vi "Single Tone Measurements.vi"() -> ()   [LabVIEW 2022 SP3]
uses:
  <vilib>/PDM Acquisition Toolkit/host/Classes/Session/Controls/Logic Levels.ctl
  <vilib>/PDM Acquisition Toolkit/shared/controls/decimation order.ctl
  source/shared/measurements/controls/single tone microphone measurements.ctl
  <vilib>/addons/_NISVFA/_Generation/Signal Generation/SV Signal/sv_System Timing Model.ctl
  <vilib>/PDM Acquisition Toolkit/host/Classes/Tasks/PDM Tasks/Controls/Acquisition Mode.ctl
  <vilib>/PDM Acquisition Toolkit/shared/controls/clock mode.ctl
  <vilib>/PDM Acquisition Toolkit/host/API/Controls/PDM Digital Start Trigger Cluster.ctl
  <vilib>/PDM Acquisition Toolkit/shared/controls/PXI trigger lines.ctl
  <vilib>/PDM Acquisition Toolkit/shared/controls/trigger polarity.ctl
  source/shared/Stop Variable Action.ctl
  source/shared/measurements/controls/audio filter settings.ctl
  class-d-amplifier/source/shared/controls/weighting filter.ctl
  class-d-amplifier/source/shared/controls/highpass filter.ctl
  class-d-amplifier/source/shared/controls/lowpass filter.ctl
  source/shared/measurements/controls/units settings - mic.ctl
  source/shared/measurements/controls/measurement units.ctl
  source/shared/measurements/controls/single tone microphone measurement settings.ctl
  <vilib>/DAQmx/read.llb/DAQmx Read (Analog Wfm 1Chan NSamp).vi
  <vilib>/DAQmx/write.llb/DAQmx Write (Analog Wfm 1Chan NSamp).vi
  <vilib>/addons/_NISVFA/_Generation/Signal Generation/SV Sinusoid/SV Sinusoid.lvclass
  C:/Program Files/NI/LVAddons/nisvt/1/vi.lib/addons/_NISVFA/_Generation/Signal Generation/SV Signal/SV Signal.lvclass
  <vilib>/PDM Acquisition Toolkit/host/API/Public/Create Tasks/Create PDM Input Task.vi
  <vilib>/PDM Acquisition Toolkit/host/API/Public/Configure/Timing/Configure Timing - PDM Input.vi
  <vilib>/PDM Acquisition Toolkit/host/API/Public/Configure/PDM Channel/Configure Microphone Sensitivity DBFS.vi
  <vilib>/PDM Acquisition Toolkit/host/API/Public/Configure/Triggering/Configure PDM Trigger (Digital Edge).vi
  <vilib>/PDM Acquisition Toolkit/host/API/Public/Read/Read PCM Waveform.vi
  <vilib>/Waveform/WDTOps.llb/WDT Waveform Duration DBL.vi
  <vilib>/Waveform/WDTOps.llb/WDT Get Waveform Subset DBL.vi
  <vilib>/addons/_NISVFA/_Generation/Signal Generation/SV Sinusoid/Configure Sine.vi
  <vilib>/DAQmx/create/channels.llb/DAQmx Create Channel (AO-Voltage-Basic).vi
  <vilib>/DAQmx/configure/timing.llb/DAQmx Timing (Sample Clock).vi
  <vilib>/DAQmx/configure/events/hardwareSignals.llb/DAQmx Export Signal (Most Signals).vi
  <vilib>/addons/_NISVFA/_Generation/Signal Generation/SV Signal/Write Sample Rate.vi
  <vilib>/addons/_NISVFA/_Generation/Signal Generation/SV Signal/Write System Timing Model.vi
  <vilib>/addons/_NISVFA/_Generation/Signal Generation/SV Signal/Write Ramp Parameters.vi
  <vilib>/DAQmx/create/channels.llb/DAQmx Create Channel (AI-Sound Pressure-Microphone).vi
  <vilib>/DAQmx/configure/trigger.llb/DAQmx Start Trigger (Digital Edge).vi
  <vilib>/DAQmx/miscellaneous.llb/DAQmx Fill In Error Info.vi
  <vilib>/addons/Sound and Vibration/svt_Level/SVL Leq Sound Level (1 Ch).vi
  <vilib>/PDM Acquisition Toolkit/host/API/Public/Clear/Clear PDM Input Task.vi
  <vilib>/addons/_NISVFA/_Generation/Signal Generation/SV Signal/SV Signal.lvclass
  <resource>/objmgr/daqmx.rc
  <vilib>/addons/Sound and Vibration/svt_Level/SoundVib_SoundLevel.lvlib
  <vilib>/PDM Acquisition Toolkit/host/API/PDM Acquisition Toolkit.lvlib
  <vilib>/PDM Acquisition Toolkit/host/Classes/Tasks/PDM Tasks/PDM Task.lvclass
  <vilib>/PDM Acquisition Toolkit/shared/PDM Shared.lvlib
  <vilib>/PDM Acquisition Toolkit/host/Classes/Session/DecoderSession.lvclass
panel:
  out "measurements":T1
  in  "Tab Control":enum32{"Time Domain", "Spectrum"}(tab)
  out "Waveform Graph":waveform(dbl)[](graph)
  out "Spectrum":cluster{"x0":dbl, "dx":dbl, "magnitude":dbl[]}[](graph)
  out "microphone sensitivity (dBFS)":dbl
  out "Ref Mic Sound Level":dbl format="%.2f"
  out "Error Out":errorcluster
  out "Actual PCM Clock Rate":dbl=47999.99987881165 format="%#_6p"
  out "Actual PDM Clock Rate":dbl=3071999.9922439456 format="%#_6p"
  out "Digital Mic Sound Level":dbl=102.39991597507856 format="%.2f"
  in  "Microphone Sensitivity (dBFS)":dbl=-26.0 format="%#_13g"
  in  "PDM Clock Rate":dbl=3072000.0 format="%#_6p"
  in  "Decimation Factor":T2=64 items=["24"=24, "32"=32, "48"=48, "64"=64, "96"=96, "128"=128]
  in  "Logic Level":T3
  in  "PDM Channels":string="PXI1Slot5\\PDMi 0"
  in  "output voltage ratio":dbl=3.39 format="%#_g Pa/V"
  in  "amplitude":dbl=94.0 format="%.2p dBSPL"
  in  "sensor sensitivity [mV/Pa]":dbl=50.0
  in  "physical channel":tag="PXI1Slot2/ai0"
  in  "output channels":tag="PXI1Slot2/ao0"
  in  "frequency":dbl=1000.0 format="%#_g Hz"
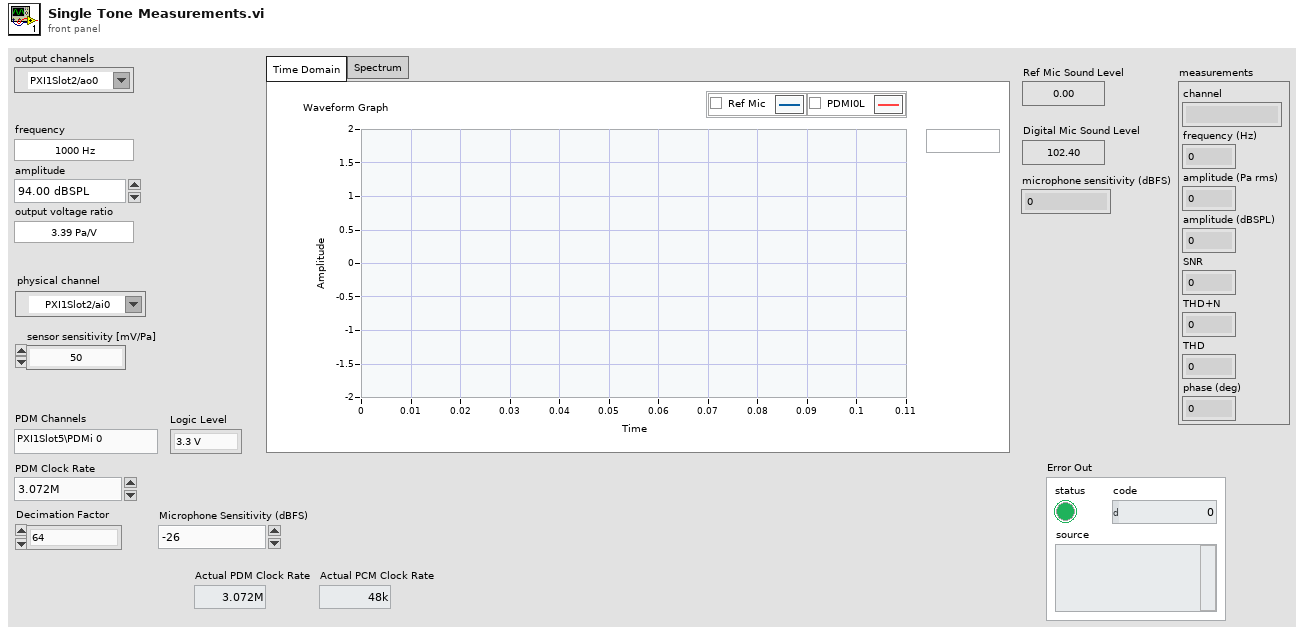
[diagram p1: front panel]
types:
  T1 = typedef "single tone microphone measurements.ctl" = cluster{"channel":string, "frequency (Hz)":dbl, "amplitude (Pa rms)":dbl, "amplitude (dBSPL)":dbl, "SNR":dbl, "THD+N":dbl, "THD":dbl, "phase (deg)":dbl}
  T2 = typedef "PDM Shared.lvlib/decimation order.ctl" = u16
  T3 = typedef "PDM Acquisition Class Library.lvlib/DecoderSession.lvclass/Logic Levels.ctl" = enum16{"3.3 V", "1.8 V", "1.2 V"}
  T4 = typedef "single tone microphone measurement settings.ctl" = cluster{"Band start":dbl, "Band stop":dbl, "Frequency":dbl}
  T5 = typedef "units settings - mic.ctl" = cluster{"SNR units":T6, "THD+N units":T6, "THD units":T6}
  T6 = typedef "measurement units.ctl" = enum32{"dB", "%", "x/y"}
  T7 = typedef "audio filter settings.ctl" = cluster{"weighting filter":T8, "highpass filter":T9, "lowpass filter ":T10}
  T8 = typedef "weighting filter.ctl" = enum32{"Linear", "A-weighting", "B-weighting", "C-weighting"}
  T9 = typedef "highpass filter.ctl" = enum32{"DC", "AC"}
  T10 = typedef "lowpass filter.ctl" = enum32{"No filter", "AES17 20kHz", "AES17 40kHz"}
  T11 = typedef "Stop Variable Action.ctl" = enum16{"Reset", "Check", "Stop"}
  T12 = typedef "PDM Acquisition Toolkit.lvlib/PDM Digital Start Trigger Cluster.ctl" = cluster{"source":T13, "polarity":T14}
  T13 = typedef "PDM Shared.lvlib/PXI trigger lines.ctl" = enum16{"PXI_Trig0", "PXI_Trig1", "PXI_Trig2", "PXI_Trig3", "PXI_Trig4", "PXI_Trig5", "PXI_Trig6", "PXI_Trig7"}
  T14 = typedef "PDM Shared.lvlib/trigger polarity.ctl" = enum16{"Rising Edge", "Falling Edge"}
  T15 = typedef "PDM Shared.lvlib/clock mode.ctl" = enum16{"divided clock", "DDS"}
  T16 = typedef "PDM Acquisition Class Library.lvlib/PDM Task.lvclass/Acquisition Mode.ctl" = enum16{"Finite", "Continuous"}
  T17 = typedef "SV Signal.lvclass/sv_System Timing Model.ctl" = i64
  T18 = cluster{"profile":enum16{"Linear", "Half cosine"}, "durations [s]":cluster{"ramp-up":dbl, "transition":dbl, "ramp-down":dbl}}
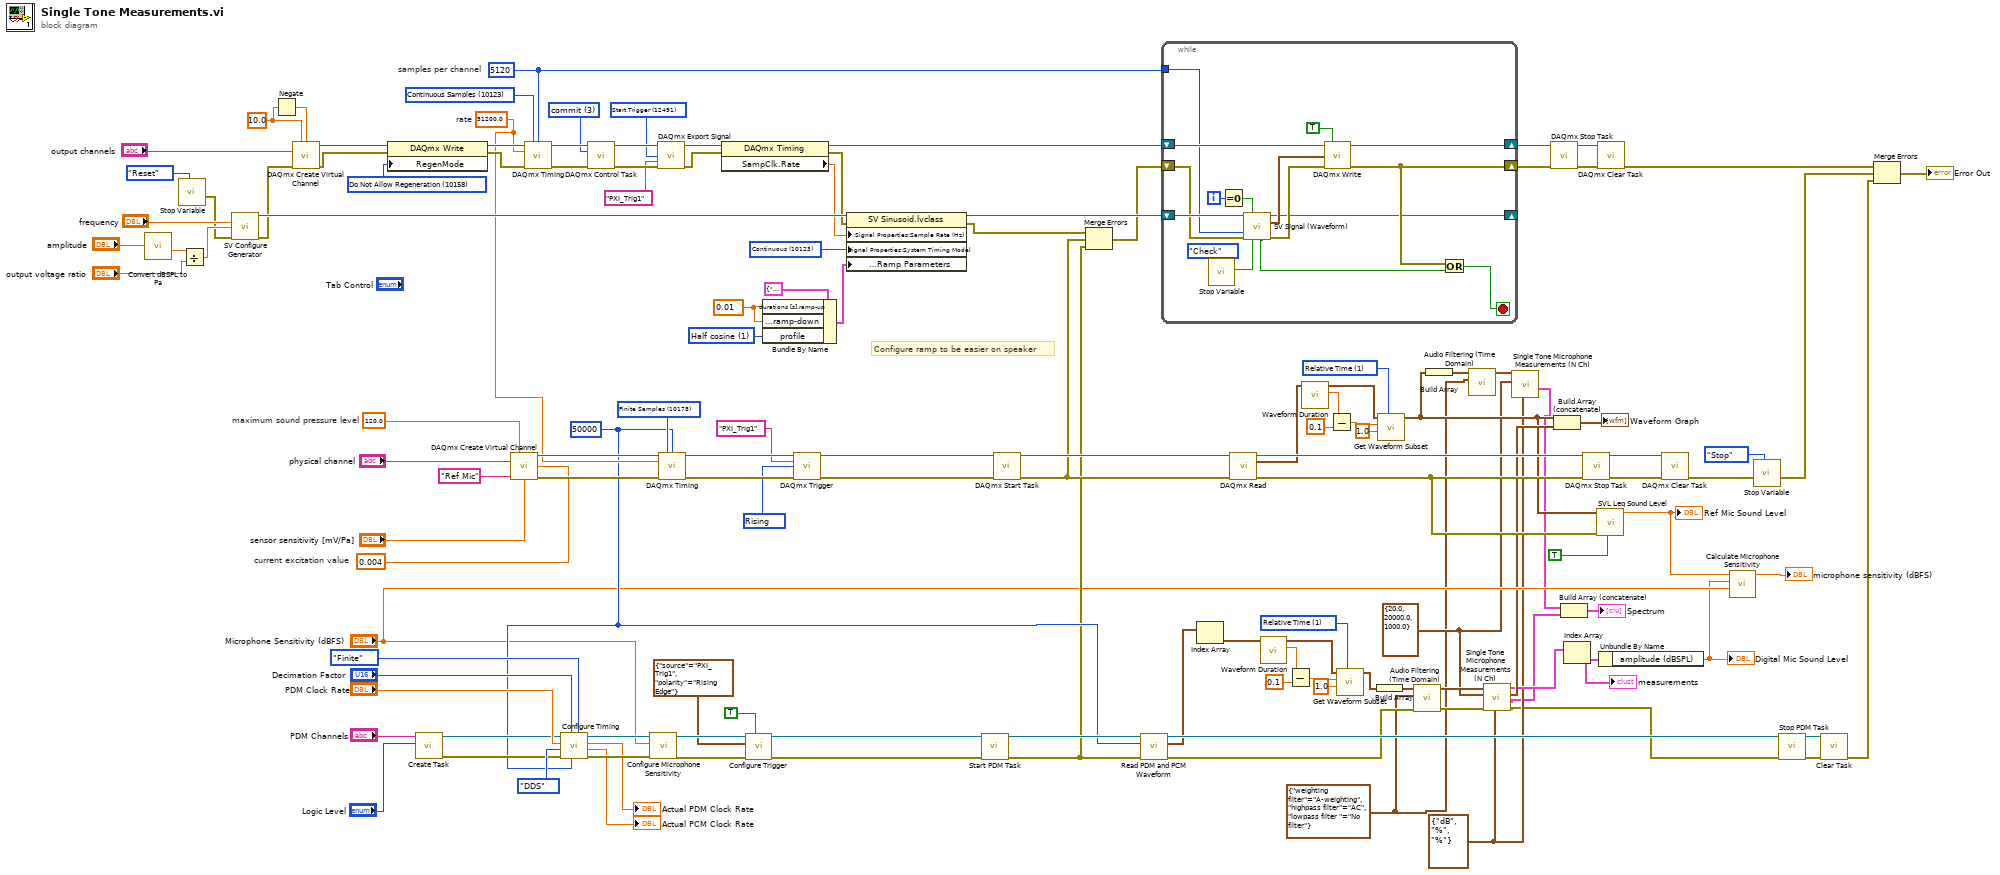
[diagram p0: block diagram]
diagram:
  w7 = T4 {"Band start"=20.0, "Band stop"=20000.0, "Frequency"=1000.0} ("measurement settings")
  w5 = T5 {"SNR units"=enum."dB", "THD+N units"=enum."%", "THD units"=enum."%"} ("units settings")
  w6 = T7 {"weighting filter"=enum."A-weighting", "highpass filter"=enum."AC", "lowpass filter "=enum."No filter"} ("filter settings")
  w38 = u16 1 items=["Samples", "Relative Time"] ("start/duration format")
  w44 = u16 1 items=["Samples", "Relative Time"] ("start/duration format")
  w61 = 50000 ("samples per channel")
  w62 = 10280 items=["Rising"=10280, "Falling"=10171] ("edge")
  w69 = 12491 items=["AI Convert Clock"=12484, "10MHz Reference Clock"=12536, "20MHz Timebase Clock"=12486, "Sample Clock"=12487, "Advance Trigger"=12488, "Reference Trigger"=12490, "Start Trigger"=12491, "Advance Complete Event"=12492, "AI Hold Complete Event"=12493, "Counter Output Event"=12494, "Change Detection Event"=12511, "Watchdog Timer Expired Event"=12512] ("signal")
  w74 = 3 items=["verify"=2, "reserve"=4, "commit"=3, "unreserve"=5, "abort"=6] ("action")
  w131 = 0.01 ("ramp duration")
  w129 = u16 1 items=["Linear", "Half cosine"] ("ramp profile")
  w109 = 0.004  # current excitation value
  w113 = 120.0  # maximum sound pressure level
  w115 = 10178 items=["Finite Samples"=10178, "Continuous Samples"=10123] ("sample mode")
  w122 = 10158 items=["Allow Regeneration"=10097, "Do Not Allow Regeneration"=10158] ("RegenMode")
  w125 = 10.0 ("maximum value")
  w102 = 5120  # samples per channel
  w126 = 10123 items=["Finite Samples"=10178, "Continuous Samples"=10123, "Hardware Timed Single Point"=12522] ("sample mode")
  w105 = 51200.0  # rate
  w128 = T17 10123 items=["Finite"=10178, "-"=-1, "Continuous"=10123, "-"=-2, "Settled"=110123, "Averaged"=210123, "Discrete Sweep"=310123, "Continuous Sweep"=410123] ("System Timing Model")
  # "Configure ramp to be easier on speaker"
  n1 = call "Convert dBSPL to Pa.vi"("dB SPL"="amplitude") -> ("Pa pk"=w95:dbl)  [unwired: 9 in, 1 out]
  n2 = call "Stop Variable.vi"("action"=Stop_Variable_Action."Reset") -> ("error out"=w35:errorcluster)  [unwired: 9 in, 1 out]
  n3 = Divide(x=w95, y="output voltage ratio") -> (x/y=w94:dbl)
  n4 = call-poly <vilib>:"SV Configure Generator.vi"("frequency (Hz)"="frequency", "amplitude"=w94, "error in (no error)"=w35) -> ("signal configuration"=w133:refnum<class "SV Sinusoid.lvclass">, "error out"=w123:errorcluster)  [unwired: 11 in]
  n5 = Negate(x=w125) -> (-x=w124:dbl)
  n6 = call-poly <vilib>:"DAQmx Create Virtual Channel.vi"("maximum value"=w125, "minimum value"=w124, "physical channels"="output channels", "error in"=w123) -> ("task out"=w121:refnum<k21>, "error out"=w119:errorcluster)  [unwired: 10 in]
  n7 = property class="DAQmx Write"(reference=w121, error in=w119, "RegenMode"=w122) -> (reference out=w120:refnum<k21>, error out=w118:errorcluster)
  n8 = call-poly <vilib>:"Create Task.vi"("logic level"="Logic Level", "channel list"="PDM Channels") -> ("error out"=w80:errorcluster, "PDM input task out"=w81:refnum<data-value>)  [unwired: 8 in]
  n9 = call-poly <vilib>:"DAQmx Create Virtual Channel.vi"("maximum sound pressure level"=w113, "physical channels"="physical channel", "name to assign"="Ref Mic", "current excitation value"=w109, "microphone sensitivity"="sensor sensitivity [mV/Pa]") -> ("task out"=w111:refnum<k21>, "error out"=w110:errorcluster)  [unwired: 9 in]
  n10 = call-poly <vilib>:"DAQmx Timing.vi"("task/channels in"=w120, "sample mode"=w126, "samples per channel"=w102, "rate"=w105, "error in"=w118) -> ("task out"=w76:refnum<k21>, "error out"=w75:errorcluster)  [unwired: 9 in]
  n11 = call-poly <vilib>:"Configure Timing.vi"("acquisition mode"=Acquisition_Mode."Finite" ("Acquisition Mode"), "number of PCM samples"=w61, "decimation factor"="Decimation Factor", "error in"=w80, "clock mode"=clock_mode."DDS" ("Clock Type"), "PDM clock rate"="PDM Clock Rate", "PDM input task in"=w81) -> ("error out"=w84:errorcluster, "actual PCM clock rate"=→"Actual PCM Clock Rate":dbl, "actual PDM clock rate"=→"Actual PDM Clock Rate":dbl, "PDM input task out"=w85:refnum<data-value>)  [unwired: 1 in]
  n12 = call <vilib>:"DAQmx Control Task.vi"("task/channels in"=w76, "action"=w74, "error in"=w75) -> ("task out"=w73:refnum<k21>, "error out"=w72:errorcluster)  [unwired: 11 in]
  n13 = call-poly <vilib>:"Configure Microphone Sensitivity.vi"("error in"=w84, "microphone sensitivity (dBFS)"="Microphone Sensitivity (dBFS)", "PDM input task in"=w85) -> ("error out"=w57:errorcluster, "PDM input task out"=w60:refnum<data-value>)  [unwired: 7 in]
  n14 = call-poly <vilib>:"DAQmx Export Signal.vi"("task/channels in"=w73, "signal"=w69, "output terminal"="PXI_Trig1", "error in"=w72) -> ("task out"=w71:refnum<k21>, "error out"=w70:errorcluster)  [unwired: 10 in]
  n15 = call-poly <vilib>:"DAQmx Timing.vi"("task/channels in"=w111, "sample mode"=w115, "samples per channel"=w61, "rate"=w105, "error in"=w110) -> ("task out"=w67:refnum<k21>, "error out"=w65:errorcluster)  [unwired: 9 in]
  n16 = property class="DAQmx Timing"(reference=w71, error in=w70) -> (reference out=w108:refnum<k21>, error out=w116:errorcluster, "SampClk.Rate"=w117:dbl)
  n17 = call-poly <vilib>:"Configure Trigger.vi"("remove filter delay samples"=TRUE, "error in"=w57, "trigger configuration"=T12 {"source"=enum."PXI_Trig1", "polarity"=enum."Rising Edge"}, "PDM input task in"=w60) -> ("error out"=w58:errorcluster, "PDM input task out"=w59:refnum<data-value>)  [unwired: 6 in]
  n18 = Bundle By Name(cluster=T18 {"profile"=enum."Linear", "durations [s]"={"ramp-up"=0.0, "transition"=0.0, "ramp-down"=0.0}} ("Ramp Parameters:All Elements"), "durations [s].ramp-up"=w131, "durations [s].ramp-down"=w131, "profile"=w129) -> (w130:T18)
  n19 = call-poly <vilib>:"DAQmx Trigger.vi"("task/channels in"=w67, "source"="PXI_Trig1", "edge"=w62, "error in"=w65) -> ("task out"=w66:refnum<k21>, "error out"=w64:errorcluster)  [unwired: 10 in]
  n20 = property class="SV Sinusoid.lvclass"(reference=w133, error in=w116, "Signal Properties:Sample Rate (Hz)"=w117, "Signal Properties:System Timing Model"=w128, "Signal Properties:Ramps:Ramp Parameters"=w130) -> (reference out=w107:refnum<class "SV Sinusoid.lvclass">, error out=w54:errorcluster)
  n21 = call <vilib>:"Start PDM Task.vi"("error in"=w58, "PDM input task in"=w59) -> ("error out"=w52:errorcluster, "PDM input task out"=w89:refnum<data-value>)  [unwired: 8 in]
  n22 = call <vilib>:"DAQmx Start Task.vi"("task/channels in"=w66, "error in"=w64) -> ("task out"=w100:refnum<k21>, "error out"=w53:errorcluster)  [unwired: 12 in]
  n23 = Merge Errors(w54, w53, w52) -> (w51:errorcluster)
  n24 = call-poly <vilib>:"Read PDM and PCM Waveform.vi"("error in"=w52, "samples per channel"=w61, "PDM input task in"=w89) -> ("error out"=w19:errorcluster, "PCM waveforms"=w77:waveform(dbl)[], "PDM input task out"=w92:refnum<data-value>)  [unwired: 5 in, 1 out]
  n25 = while {
    tunnel: w102 -> [w147]
    shift-right: [w145] -> w25
    shift-left: w108 -> [w149]
    shift-right: [w146] -> w24
    shift-left: w51 -> [w141]
    shift-right: [w140] -> _
    shift-left: w107 -> [w148]
    i -> [w137]
    stop <- w139 stop-if-true
    n26 = call "Stop Variable.vi"("action"=Stop_Variable_Action."Check") -> ("stop"=w135:bool)  [unwired: 9 in, 1 out]
    n27 = Equal To 0?(x=w137) -> (x = 0?=w138:bool)
    n28 = call-dynamic "SV Signal (Waveform).vi"("signal configuration"=w148, "reset"=w138, "samples"=w147, "error in (no error)"=w141, "stop"=w135) -> ("signal configuration"=w140:refnum<class "SV Sinusoid.lvclass">, "output waveform"=w143:waveform(dbl), "done"=w136:bool, "error out"=w144:errorcluster)  [unwired: 5 in, 2 out]
    n29 = call-poly <vilib>:"DAQmx Write.vi"("task/channels in"=w149, "auto start"=TRUE, "data"=w143, "error in"=w144) -> ("task out"=w145:refnum<k21>, "error out"=w146:errorcluster)  [unwired: 9 in, 1 out]
    n30 = Or(x=w146, y=w136) -> (x .or. y?=w139:bool)
  }
  n31 = Index Array(array=w77) -> (element=w50:waveform(dbl))  [unwired: 1 in]
  n32 = call-poly <vilib>:"DAQmx Read.vi"("task/channels in"=w100, "error in"=w53) -> ("task out"=w99:refnum<k21>, "data"=w37:waveform(dbl), "error out"=w98:errorcluster)  [unwired: 11 in]
  n33 = call-poly <vilib>:"Waveform Duration.vi"("waveform in"=w50) -> ("duration"=w49:dbl, "waveform out"=w45:waveform(dbl))  [unwired: 8 in, 1 out]
  n34 = Subtract(x=w49, y=0.1) -> (x-y=w46:dbl)
  n35 = call-poly <vilib>:"Waveform Duration.vi"("waveform in"=w37) -> ("duration"=w43:dbl, "waveform out"=w39:waveform(dbl))  [unwired: 8 in, 1 out]
  n36 = Subtract(x=w43, y=0.1) -> (x-y=w40:dbl)
  n37 = call-poly <vilib>:"Get Waveform Subset.vi"("start/duration format"=w44, "duration"=1.0, "start samples/time"=w46, "waveform in"=w45) -> ("waveform out"=w17:waveform(dbl))  [unwired: 2 in, 3 out]
  n38 = Build Array(w17) -> (w18:waveform(dbl)[])
  n39 = call-poly <vilib>:"Get Waveform Subset.vi"("start/duration format"=w38, "duration"=1.0, "start samples/time"=w40, "waveform in"=w39) -> ("waveform out"=w10:waveform(dbl))  [unwired: 2 in, 3 out]
  n40 = call "Audio Filtering (Time Domain).vi"("waveforms"=w18, "filter settings"=w6, "error in"=w19) -> ("time domain"=w15:waveform(dbl)[], "error out"=w16:errorcluster)  [unwired: 6 in]
  n41 = Build Array(w10) -> (w9:waveform(dbl)[])
  n42 = call "Audio Filtering (Time Domain).vi"("waveforms"=w9, "filter settings"=w6) -> ("time domain"=w8:waveform(dbl)[])  [unwired: 7 in, 1 out]
  n43 = call "Single Tone Microphone Measurements (N Ch).vi"("units settings"=w5, "error in"=w16, "measurement settings"=w7, "waveforms"=w15) -> ("error out"=w1:errorcluster, "spectra"=w4:cluster{"x0":dbl, "dx":dbl, "magnitude":dbl[]}[], "waveforms"=w14:waveform(dbl)[], "measurements"=w13:T1[])  [unwired: 4 in]
  n44 = call "Single Tone Microphone Measurements (N Ch).vi"("units settings"=w5, "measurement settings"=w7, "waveforms"=w8) -> ("spectra"=w3:cluster{"x0":dbl, "dx":dbl, "magnitude":dbl[]}[])  [unwired: 5 in, 3 out]
  n45 = call <vilib>:"DAQmx Stop Task.vi"("task/channels in"=w25, "error in"=w24) -> ("task out"=w23:refnum<k21>, "error out"=w22:errorcluster)  [unwired: 12 in]
  n46 = Build Array (concatenate)(w10, w14) -> (→"Waveform Graph":waveform(dbl)[])
  n47 = Build Array (concatenate)(w3, w4) -> (→"Spectrum":cluster{"x0":dbl, "dx":dbl, "magnitude":dbl[]}[])
  n48 = Index Array(array=w13) -> (element=w12:T1)  [unwired: 1 in]
  "measurements" <- w12
  n49 = call <vilib>:"DAQmx Stop Task.vi"("task/channels in"=w99, "error in"=w98) -> ("task out"=w106:refnum<k21>, "error out"=w103:errorcluster)  [unwired: 12 in]
  n50 = call-poly <vilib>:"SVL Leq Sound Level.vi"("restart averaging (F)"=TRUE, "error in (no error)"=w98, "scaled signal [EU]"=w10) -> ("Leq sound level [dB EU]"=w31:dbl)  [unwired: 6 in, 2 out]
  "Ref Mic Sound Level" <- w31
  n51 = call <vilib>:"DAQmx Clear Task.vi"("task in"=w23, "error in"=w22) -> ("error out"=w21:errorcluster)  [unwired: 13 in]
  n52 = Unbundle By Name(w12) -> ("amplitude (dBSPL)"=w11:dbl)
  "Digital Mic Sound Level" <- w11
  n53 = call <vilib>:"DAQmx Clear Task.vi"("task in"=w106, "error in"=w103) -> ("error out"=w32:errorcluster)  [unwired: 13 in]
  n54 = call "Calculate Microphone Sensitivity.vi"("microphone sensitivity (dBFS)"="Microphone Sensitivity (dBFS)", "measured sound level (dBSPL)"=w11, "reference sound level (dBSPL)"=w31) -> ("calculated microphone sensitivity (dBFS)"=→"microphone sensitivity (dBFS)":dbl)  [unwired: 8 in]
  n55 = call "Stop Variable.vi"("action"=Stop_Variable_Action."Stop", "error in (no error)"=w32) -> ("error out"=w27:errorcluster)  [unwired: 8 in, 1 out]
  n56 = call <vilib>:"Stop PDM Task.vi"("error in"=w1, "PDM input task in"=w92) -> ("error out"=w83:errorcluster, "PDM input task out"=w91:refnum<data-value>)  [unwired: 8 in]
  n57 = call-poly <vilib>:"Clear Task.vi"("error in"=w83, "PDM input task in"=w91) -> ("error out"=w26:errorcluster)  [unwired: 9 in]
  n58 = Merge Errors(w21, w27, w26) -> (→"Error Out":errorcluster)
